vi "ConfigCreateProgram.vi"(11 "singlePumpCycleRefreshRatio":dbl) -> (3 "ProgramStopped":bool)   [LabVIEW 2018, in "Config.lvlib"]
uses:
  Config.lvlib
  <vilib>/xml/NI_XML.lvlib
  <vilib>/xml/Close Reference(Node).vi
  <vilib>/xml/Load XML File.vi
panel:
  in  "error in":errorcluster
  in  "Calc Minimal Acqu time":bool
  out "Minimal Acquisition Time":timestamp format="%<%H:%M:%S%3u>T"
  in  "stop":bool
  out "Loop Microscope Settings":string[][](array[string])
  out "Positions":string[][](array[string])
  out "Micro Ok?":bool
  out "Pos Ok?":bool
  in  "Load Microscope Settings":path
  in  "Load Positions":path
  in  "Acquire":bool
  in  "Load old Prog":bool
  out "error out":errorcluster
  in  "Clear":bool
  in  "Save":bool
  in  "Loop End":bool
  in  "Loop Start":bool
  in  "Incubate":bool
  in  "Change Reagent":bool
  in  "Feed":bool
  in  "Pump":bool
  out "Program Steps":i32[](listbox)
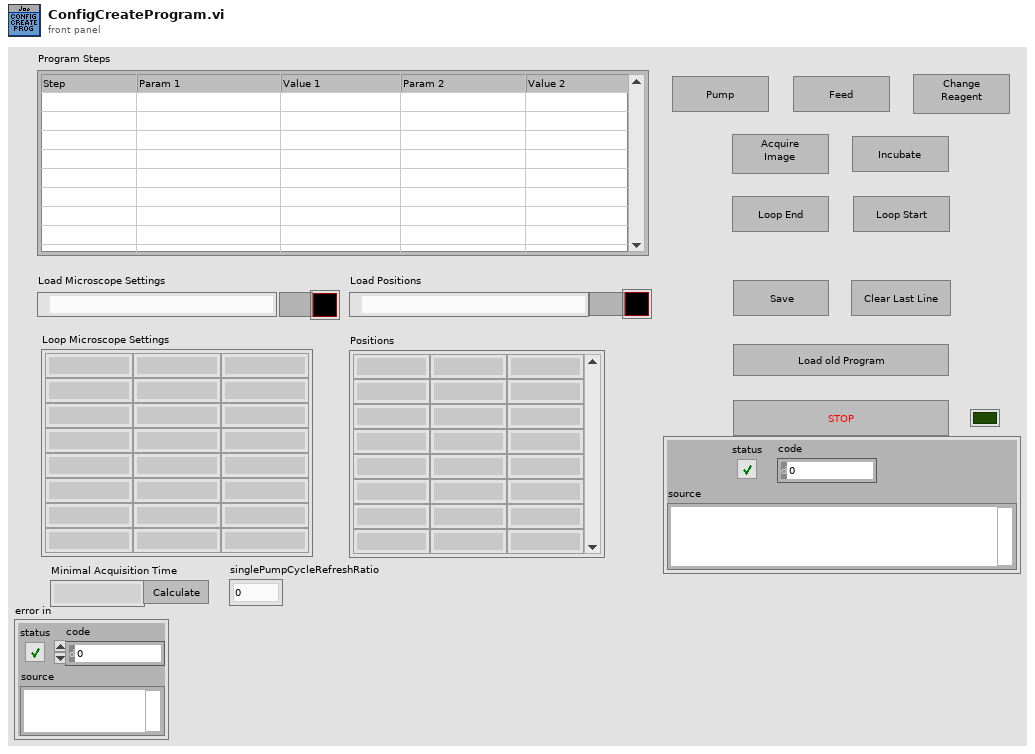
[diagram p1: front panel]
types:
  T1 = enum16{"open", "replace", "create", "open or create", "replace or create", "replace or create with confirmation"}
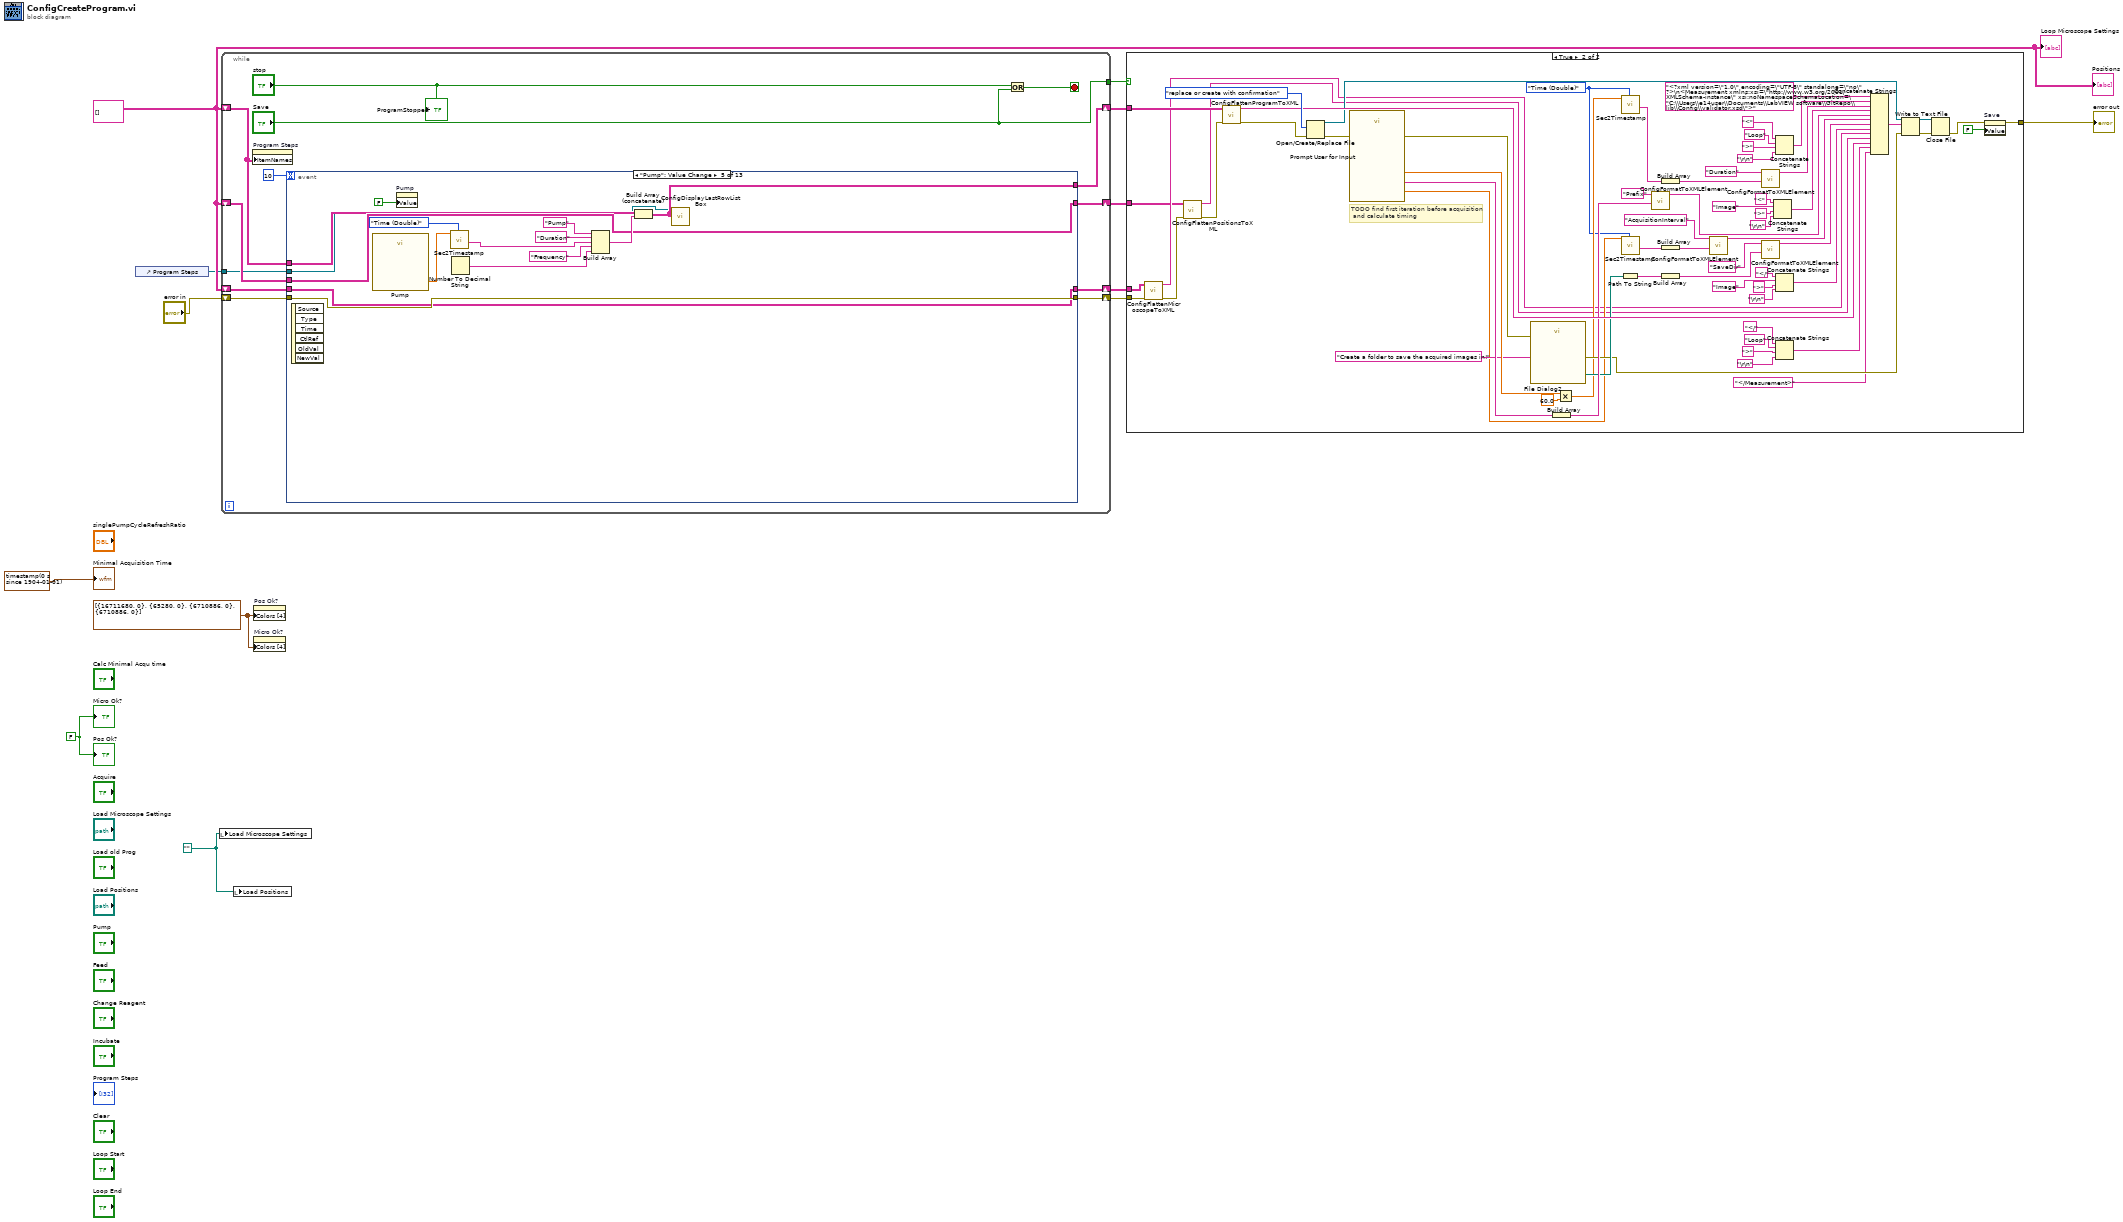
[diagram p0: block diagram]
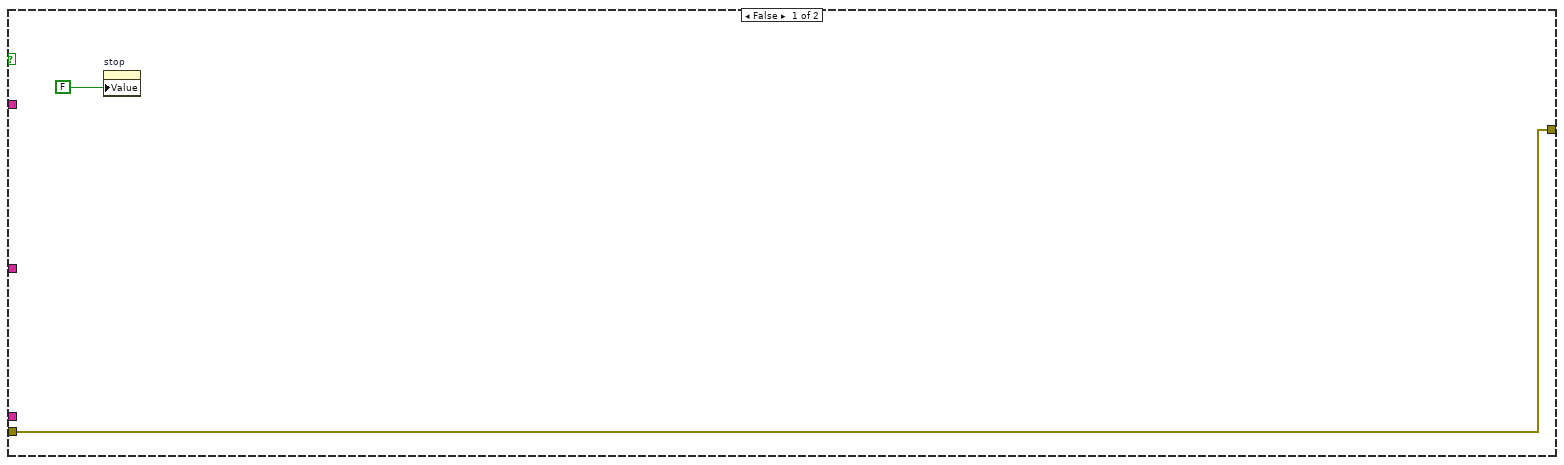
[diagram p2: hidden frame]
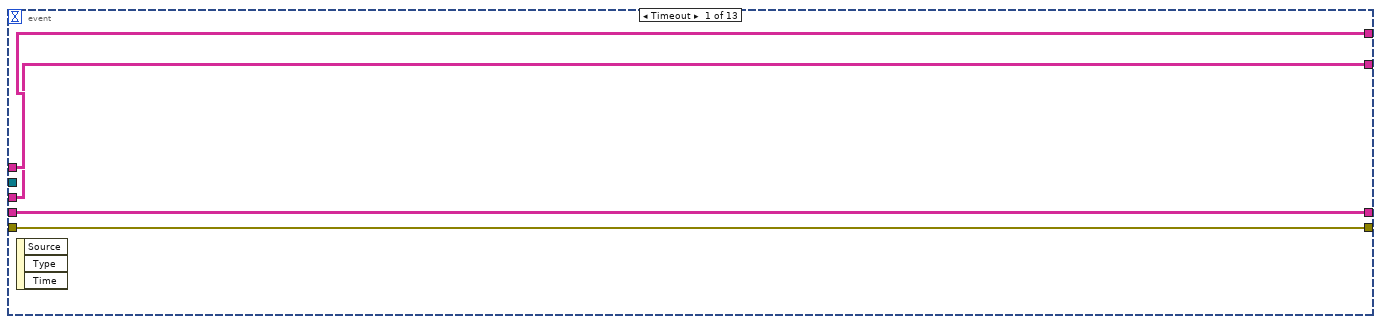
[diagram p3: hidden frame]
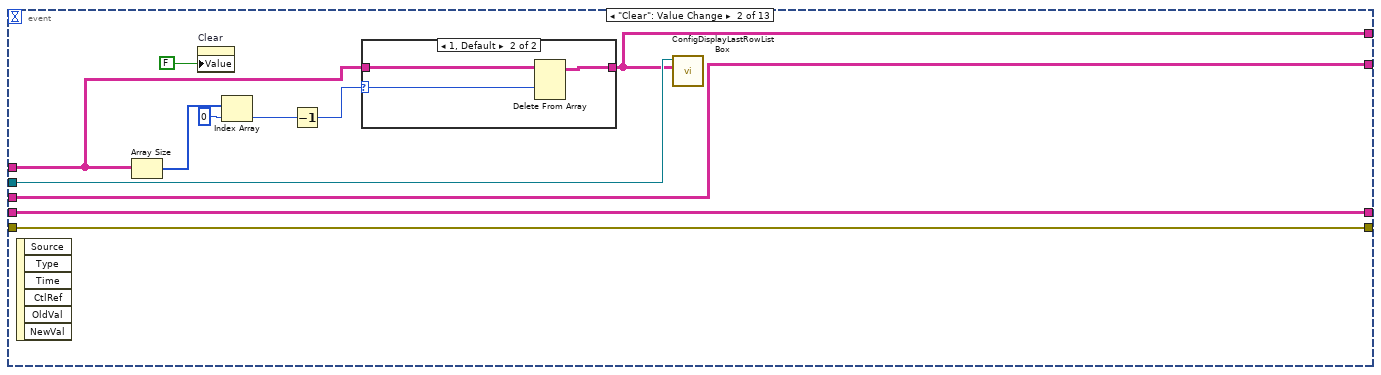
[diagram p4: hidden frame]
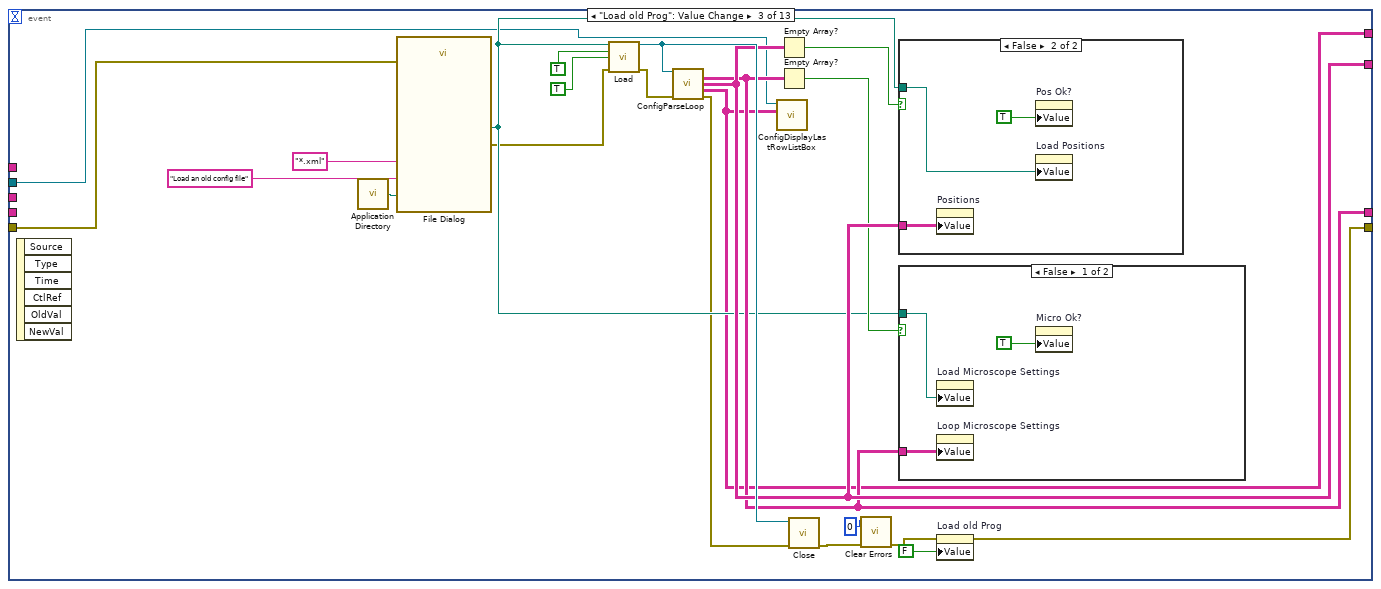
[diagram p6: hidden frame]
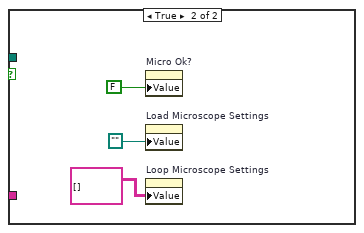
[diagram p7: hidden frame]
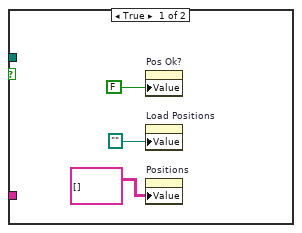
[diagram p8: hidden frame]
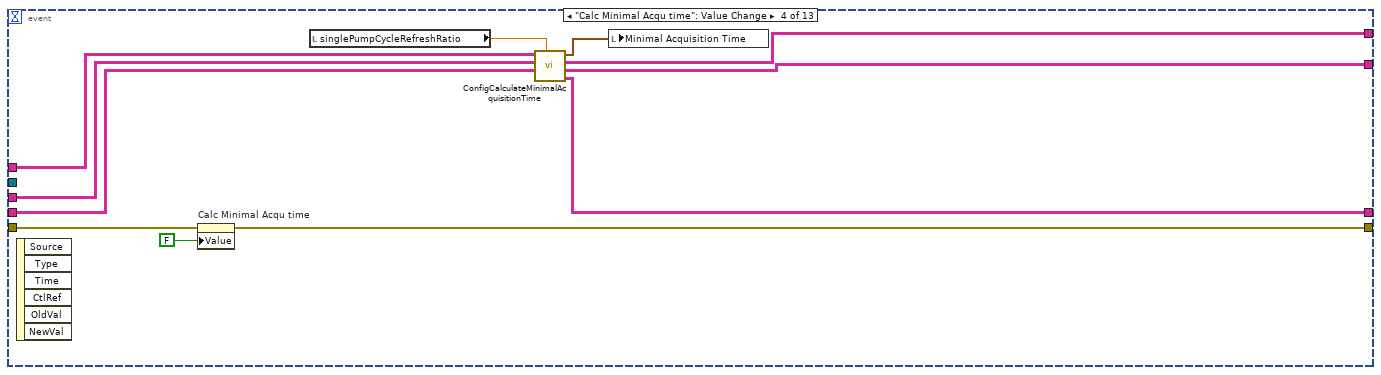
[diagram p9: hidden frame]
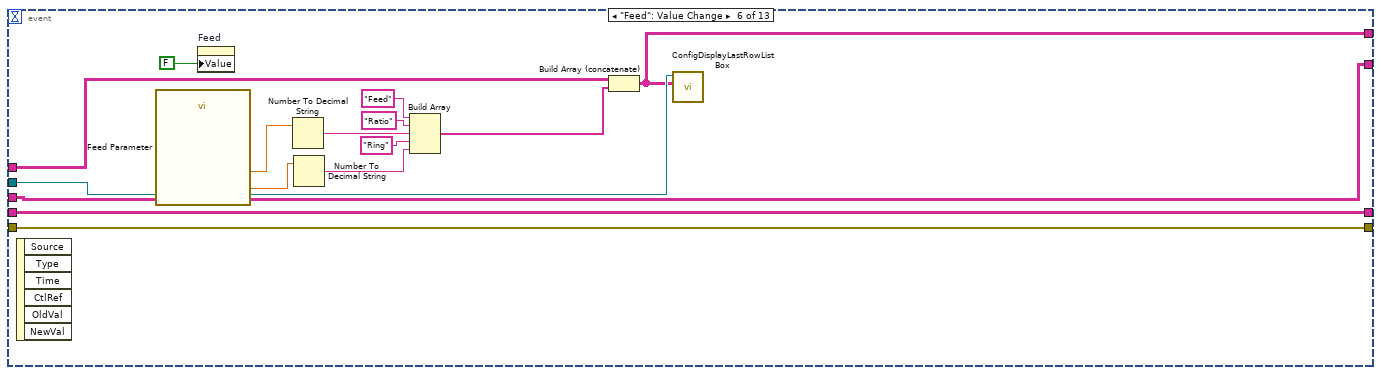
[diagram p10: hidden frame]
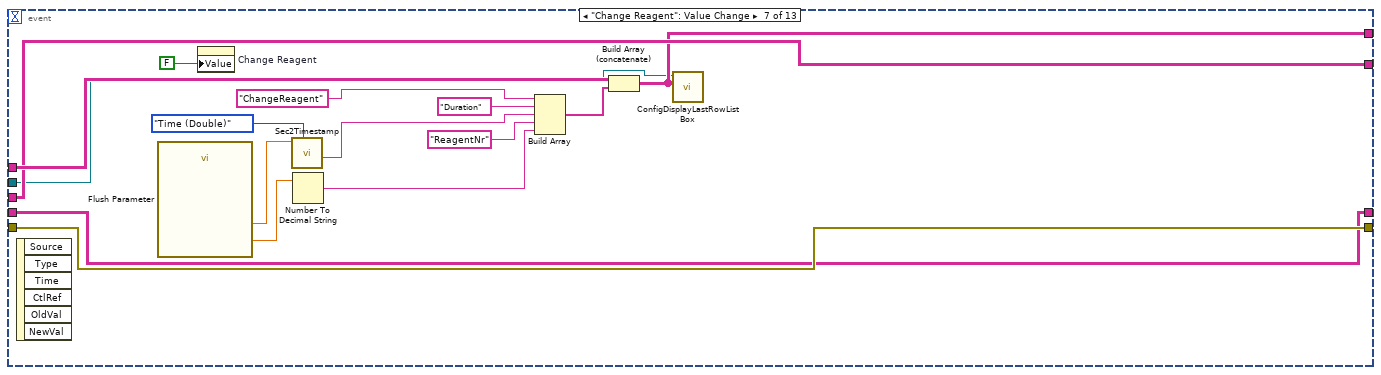
[diagram p11: hidden frame]
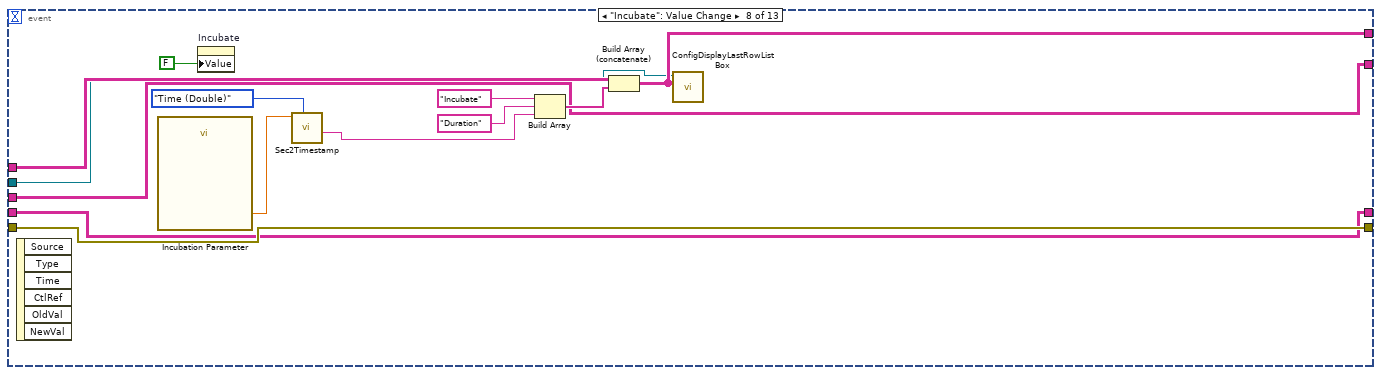
[diagram p12: hidden frame]
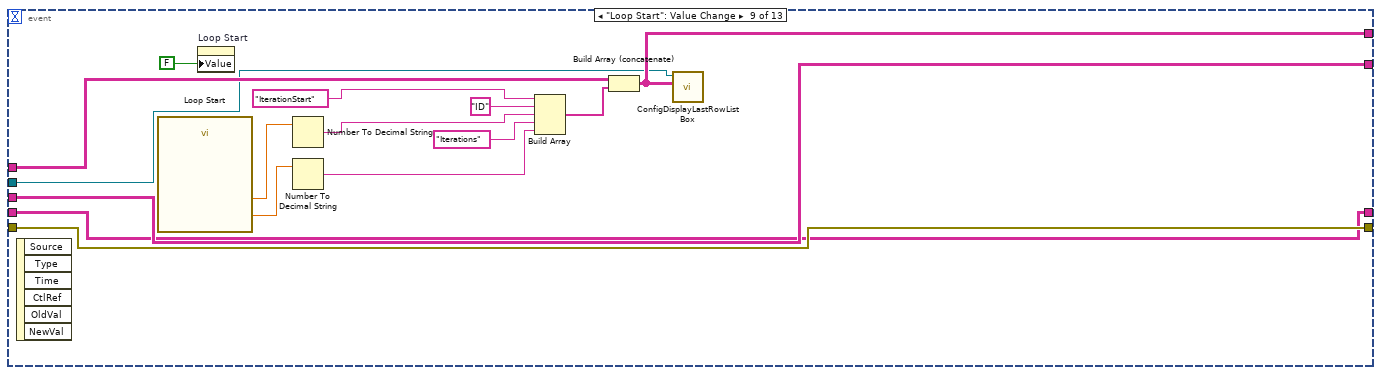
[diagram p13: hidden frame]
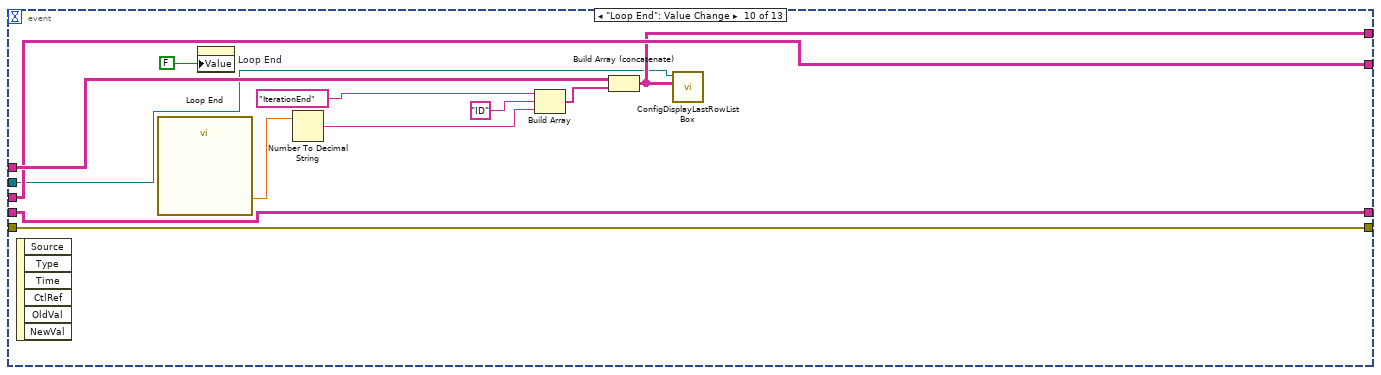
[diagram p14: hidden frame]
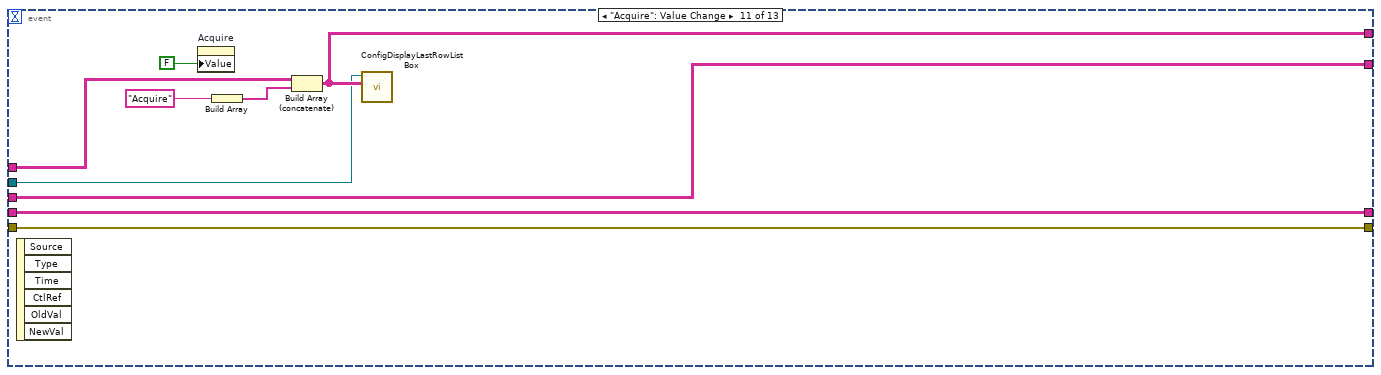
[diagram p15: hidden frame]
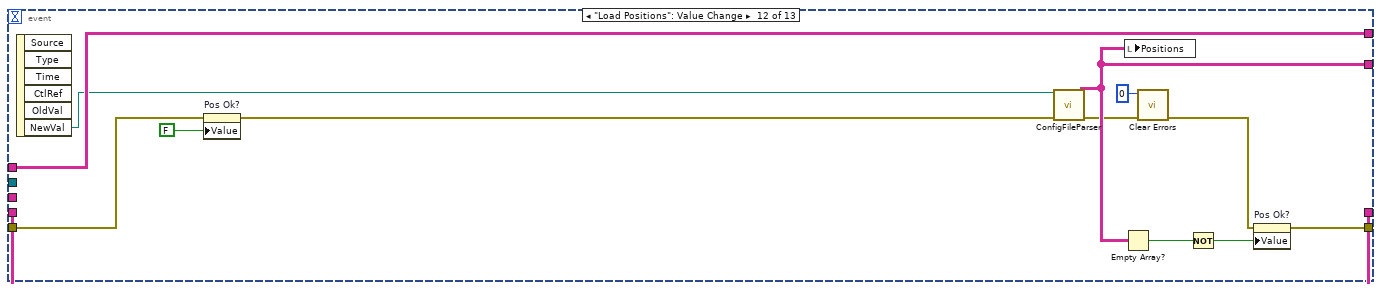
[diagram p16: hidden frame]
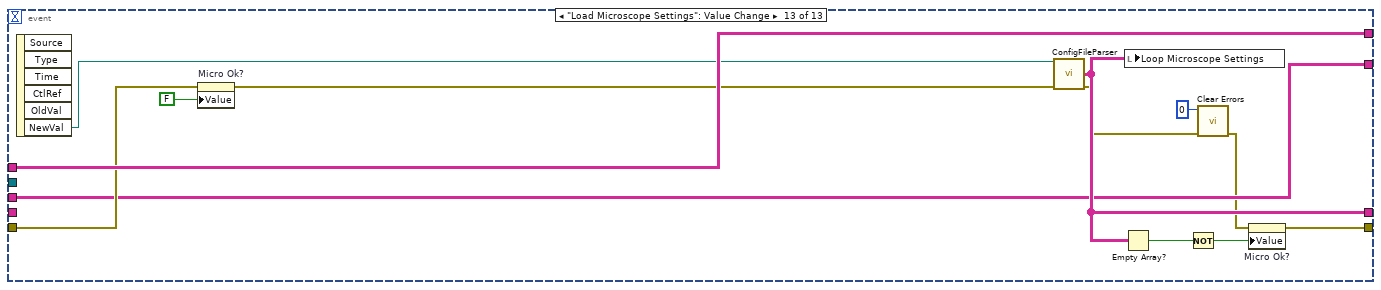
[diagram p17: hidden frame]
diagram:
  w2 = FALSE
  w3 = path ""
  w6 = string[][] [] ("ItemNames")
  w11 = cluster{u32, u32}[] [{16711680, 0}, {65280, 0}, {6710886, 0}, {6710886, 0}] ("Colors [4]")
  n1 = control-ref of="Program Steps"() -> (w5:refnum<vi>)
  n2 = local write "Load Microscope Settings"(w3) -> ()
  n3 = while {
    shift-right: [w26] -> w12
    shift-left: w6 -> [w22]
    shift-right: [w23] -> w9
    shift-left: "error in" -> [w24]
    shift-right: [w19] -> w7
    shift-left: w6 -> [w18]
    shift-right: [w20] -> w10
    shift-left: w6 -> [w21]
    tunnel: ["Save"] -> w8
    tunnel: w5 -> [w14]
    stop <- w17 stop-if-true
    n4 = property on="Program Steps" class="MCListbox (strict)"("ItemNames"=w22) -> ()  [unwired: 2 in, 2 out]
    n5 = event shown="[4] \"Pump\": Value Change" {
      selector: _ -> [_ _ _ _ _ _ _ _ _ _ _ _ _]
      dyn-events: _ -> [_ _ _ _ _ _ _ _ _ _ _ _ _]
      timeout: 10 -> [_ _ _ _ _ _ _ _ _ _ _ _ _]
      tunnel: w22 -> [w30 w41 _ w85 w95 w117 w133 w147 w161 w174 w185 w198 w211]
      tunnel: [w30 w31 w52 w80 w92 w109 w122 w138 w151 w166 w178 w198 w211] -> w26
      tunnel: w24 -> [w29 w35 w61 w88 w99 w113 w128 w144 w154 w169 w181 w193 w206]
      tunnel: [w29 w35 w54 w90 w99 w113 w128 w144 w154 w169 w181 w192 w205] -> w23
      tunnel: [w28 w34 w58 w81 w98 w112 w127 w143 w153 w168 w180 w191 w203] -> w19
      tunnel: w21 -> [w27 w33 _ w83 w97 w111 w126 w142 w152 w167 w179 w190 _]
      tunnel: [w27 w33 w56 w82 w97 w111 w126 w142 w152 w167 w179 w190 w204] -> w20
      tunnel: w18 -> [w28 w34 _ w84 w98 w112 w127 w143 w153 w168 w180 _ w203]
      tunnel: w14 -> [_ w32 w53 _ w91 w110 w121 w137 w150 w165 w177 _ _]
      event Timeout {
        n6 = event-data() -> ()  [unwired: 1 in, 3 out]
      }
      event "Clear": Value Change {
        n7 = event-data() -> ()  [unwired: 1 in, 6 out]
        n8 = Array Size(array=w41) -> (size(s)=w40:i32[])
        n9 = property on="Clear" class="Bool (strict)"("Value"=FALSE ("Value (Signaling)")) -> ()  [unwired: 2 in, 2 out]
        n10 = Index Array(array=w40, index=0) -> (element=w38:i32)
        n11 = Decrement(x=w38) -> (x-1=w37:i32)
        n12 = case shown="1, Default" w37 {
          selector: w37 -> [_ w43]
          tunnel: [w42 w45] -> w31
          tunnel: w41 -> [w42 w44]
          frame -1 {
          }
          frame 1, Default {
            n13 = Delete From Array(array=w44, index (row)=w43) -> (array with subset deleted=w45:string[][])  [unwired: 2 in, 1 out]
          }
        }
        n14 = call "ConfigDisplayLastRowListBox.vi"("Array"=w31, "reference"=w32) -> ()  [unwired: 10 in]
      }
      event "Load old Prog": Value Change {
        n15 = event-data() -> ()  [unwired: 1 in, 6 out]
        n16 = call <vilib>:"Application Directory.vi"() -> ("Application Directory"=w64:path)
        n17 = call "File Dialog"("start path"=w64, "prompt"="Load an old config file", "error in"=w61, "pattern label"="*.xml") -> ("selected path"=w55:path, "error out"=w49:errorcluster)  [unwired: 8 in, 2 out]
        n18 = call-poly <vilib>:"Load.vi"("path to XML document"=w55, "process namespaces (False)"=TRUE, "process schema (False)"=TRUE, "error in (no error)"=w49) -> ("DOM document out"=w60:refnum<k20>, "error out"=w50:errorcluster)  [unwired: 9 in, 1 out]
        n19 = call "ConfigParseLoop.vi"("Root Refnum in"=w60, "error in (no error)"=w50) -> ("Loop Microscope Settings"=w56:string[][], "Position Settings"=w58:string[][], "Program"=w52:string[][], "error out"=w51:errorcluster)  [unwired: 9 in, 1 out]
        n20 = call "ConfigDisplayLastRowListBox.vi"("Array"=w52, "reference"=w53) -> ()  [unwired: 10 in]
        n21 = Empty Array?(array=w58) -> (empty?=w59:bool)
        n22 = Empty Array?(array=w56) -> (empty?=w57:bool)
        n23 = call-poly <vilib>:"Close.vi"("error in (no error)"=w51, "node"=w60) -> ("error out"=w47:errorcluster)  [unwired: 7 in]
        n24 = call <vilib>:"Clear Errors.vi"("error in (no error)"=w47, "specific error code to clear (0: all)"=0) -> ("error out"=w46:errorcluster)  [unwired: 4 in, 1 out]
        n25 = case shown="False" w59 {
          tunnel: w58 -> [_ w79]
          tunnel: w55 -> [_ w78]
          frame True {
            n26 = property on="Pos Ok?" class="Bool (strict)"("Value"=FALSE ("Pos Ok?")) -> ()  [unwired: 2 in, 2 out]
            n27 = property on="Load Positions" class="Path"("Value"=path "") -> ()  [unwired: 2 in, 2 out]
            n28 = property on="Positions" class="Arr (strict)"("Value"=string[][] []) -> ()  [unwired: 2 in, 2 out]
          }
          frame False {
            n29 = property on="Positions" class="Arr (strict)"("Value"=w79) -> ()  [unwired: 2 in, 2 out]
            n30 = property on="Pos Ok?" class="Bool (strict)"("Value"=TRUE ("Pos Ok?")) -> ()  [unwired: 2 in, 2 out]
            n31 = property on="Load Positions" class="Path"("Value"=w78) -> ()  [unwired: 2 in, 2 out]
          }
        }
        n32 = case shown="False" w57 {
          tunnel: w56 -> [w70 _]
          tunnel: w55 -> [w69 _]
          frame False {
            n33 = property on="Load Microscope Settings" class="Path"("Value"=w69) -> ()  [unwired: 2 in, 2 out]
            n34 = property on="Loop Microscope Settings" class="Arr (strict)"("Value"=w70) -> ()  [unwired: 2 in, 2 out]
            n35 = property on="Micro Ok?" class="Bool (strict)"("Value"=TRUE ("Micro Ok?")) -> ()  [unwired: 2 in, 2 out]
          }
          frame True {
            n36 = property on="Micro Ok?" class="Bool (strict)"("Value"=FALSE ("Micro Ok?")) -> ()  [unwired: 2 in, 2 out]
            n37 = property on="Load Microscope Settings" class="Path"("Value"=path "") -> ()  [unwired: 2 in, 2 out]
            n38 = property on="Loop Microscope Settings" class="Arr (strict)"("Value"=string[][] []) -> ()  [unwired: 2 in, 2 out]
          }
        }
        n39 = property on="Load old Prog" class="Bool (strict)"(error in=w46, "Value"=FALSE ("Value (Signaling)")) -> (error out=w54:errorcluster)  [unwired: 1 in, 1 out]
      }
      event "Calc Minimal Acqu time": Value Change {
        n40 = event-data() -> ()  [unwired: 1 in, 6 out]
        n41 = property on="Calc Minimal Acqu time" class="Bool (strict)"(error in=w88, "Value"=FALSE ("Calc Minimal Acqu time")) -> (error out=w90:errorcluster)  [unwired: 1 in, 1 out]
        n42 = local read "singlePumpCycleRefreshRatio"() -> (w86:dbl)
        n43 = call "ConfigCalculateMinimalAcquisitionTime.vi"("Single Pump Cycle Refresh Ratio"=w86, "Loop Microscope Settings"=w83, "Positions"=w84, "Program"=w85) -> ("Microscope Out"=w82:string[][], "Positions out"=w81:string[][], "Program out"=w80:string[][], "Time (Time Stamp)"=w87:timestamp)  [unwired: 4 in]
        n44 = local write "Minimal Acquisition Time"(w87) -> ()
      }
      event "Pump": Value Change {
        n45 = event-data() -> ()  [unwired: 1 in, 6 out]
        n46 = call "Pump"() -> ("Duration [s] (@ 4Hz)"=w96:dbl)  [unwired: 17 in, 2 out]
        n47 = property on="Pump" class="Bool (strict)"("Value"=FALSE ("Value (Signaling)")) -> ()  [unwired: 2 in, 2 out]
        n48 = call "Sec2Timestamp.vi"("Input Selection"=enum32{"Time (Double)", "Time (Time Stamp)"}."Time (Double)", "Input Time (Double)"=w96) -> ("time string"=w93:string)  [unwired: 7 in, 2 out]
        n49 = Number To Decimal String() -> (decimal integer string=w102:string)  [unwired: 2 in]
        n50 = Build Array("Pump", "Duration", w93, "Frequency", w102) -> (w104:string[])
        n51 = Build Array (concatenate)(w95, w104) -> (w92:string[][])
        n52 = call "ConfigDisplayLastRowListBox.vi"("Array"=w92, "reference"=w91) -> ()  [unwired: 10 in]
      }
      event "Feed": Value Change {
        n53 = event-data() -> ()  [unwired: 1 in, 6 out]
        n54 = call "Feed Parameter"() -> ("Ring"=w108:dbl, "Ratio [%]"=w119:dbl)  [unwired: 16 in, 2 out]
        n55 = property on="Feed" class="Bool (strict)"("Value"=FALSE ("Value (Signaling)")) -> ()  [unwired: 2 in, 2 out]
        n56 = Number To Decimal String(number=w119) -> (decimal integer string=w115:string)  [unwired: 1 in]
        n57 = Number To Decimal String(number=w108) -> (decimal integer string=w107:string)  [unwired: 1 in]
        n58 = Build Array("Feed", "Ratio", w115, "Ring" ("element"), w107) -> (w118:string[])
        n59 = Build Array (concatenate)(w117, w118) -> (w109:string[][])
        n60 = call "ConfigDisplayLastRowListBox.vi"("Array"=w109, "reference"=w110) -> ()  [unwired: 10 in]
      }
      event "Change Reagent": Value Change {
        n61 = event-data() -> ()  [unwired: 1 in, 6 out]
        n62 = call "Flush Parameter"() -> ("Flush Duration [s]"=w125:dbl, "Reagent Nr."=w130:dbl)  [unwired: 16 in, 2 out]
        n63 = property on="Change Reagent" class="Bool (strict)"("Value"=FALSE ("Value (Signaling)")) -> ()  [unwired: 2 in, 2 out]
        n64 = call "Sec2Timestamp.vi"("Input Selection"=enum32{"Time (Double)", "Time (Time Stamp)"}."Time (Double)", "Input Time (Double)"=w125) -> ("time string"=w123:string)  [unwired: 7 in, 2 out]
        n65 = Number To Decimal String(number=w130) -> (decimal integer string=w129:string)  [unwired: 1 in]
        n66 = Build Array("ChangeReagent", "Duration", w123, "ReagentNr", w129) -> (w134:string[])
        n67 = Build Array (concatenate)(w133, w134) -> (w122:string[][])
        n68 = call "ConfigDisplayLastRowListBox.vi"("Array"=w122, "reference"=w121) -> ()  [unwired: 10 in]
      }
      event "Incubate": Value Change {
        n69 = event-data() -> ()  [unwired: 1 in, 6 out]
        n70 = call "Incubation Parameter"() -> ("Duration [s]"=w141:dbl)  [unwired: 17 in, 2 out]
        n71 = property on="Incubate" class="Bool (strict)"("Value"=FALSE ("Value (Signaling)")) -> ()  [unwired: 2 in, 2 out]
        n72 = call "Sec2Timestamp.vi"("Input Selection"=enum32{"Time (Double)", "Time (Time Stamp)"}."Time (Double)", "Input Time (Double)"=w141) -> ("time string"=w139:string)  [unwired: 7 in, 2 out]
        n73 = Build Array("Incubate", "Duration", w139) -> (w148:string[])
        n74 = Build Array (concatenate)(w147, w148) -> (w138:string[][])
        n75 = call "ConfigDisplayLastRowListBox.vi"("Array"=w138, "reference"=w137) -> ()  [unwired: 10 in]
      }
      event "Loop Start": Value Change {
        n76 = event-data() -> ()  [unwired: 1 in, 6 out]
        n77 = call "Loop Start"() -> ("ID"=w159:dbl, "Iterations"=w163:dbl)  [unwired: 16 in, 2 out]
        n78 = property on="Loop Start" class="Bool (strict)"("Value"=FALSE ("Value (Signaling)")) -> ()  [unwired: 2 in, 2 out]
        n79 = Number To Decimal String(number=w159) -> (decimal integer string=w158:string)  [unwired: 1 in]
        n80 = Number To Decimal String(number=w163) -> (decimal integer string=w155:string)  [unwired: 1 in]
        n81 = Build Array("IterationStart", "ID" ("element"), w158, "Iterations", w155) -> (w162:string[])
        n82 = Build Array (concatenate)(w161, w162) -> (w151:string[][])
        n83 = call "ConfigDisplayLastRowListBox.vi"("Array"=w151, "reference"=w150) -> ()  [unwired: 10 in]
      }
      event "Loop End": Value Change {
        n84 = event-data() -> ()  [unwired: 1 in, 6 out]
        n85 = call "Loop End"() -> ("ID"=w172:dbl)  [unwired: 17 in, 2 out]
        n86 = property on="Loop End" class="Bool (strict)"("Value"=FALSE ("Value (Signaling)")) -> ()  [unwired: 2 in, 2 out]
        n87 = Number To Decimal String(number=w172) -> (decimal integer string=w171:string)  [unwired: 1 in]
        n88 = Build Array("IterationEnd", "ID" ("element"), w171) -> (w175:string[])
        n89 = Build Array (concatenate)(w174, w175) -> (w166:string[][])
        n90 = call "ConfigDisplayLastRowListBox.vi"("Array"=w166, "reference"=w165) -> ()  [unwired: 10 in]
      }
      event "Acquire": Value Change {
        n91 = event-data() -> ()  [unwired: 1 in, 6 out]
        n92 = property on="Acquire" class="Bool (strict)"("Value"=FALSE ("Value (Signaling)")) -> ()  [unwired: 2 in, 2 out]
        n93 = Build Array("Acquire") -> (w182:string[])
        n94 = Build Array (concatenate)(w185, w182) -> (w178:string[][])
        n95 = call "ConfigDisplayLastRowListBox.vi"("Array"=w178, "reference"=w177) -> ()  [unwired: 10 in]
      }
      event "Load Positions": Value Change {
        n96 = event-data() -> ("NewVal"=w197:path)  [unwired: 1 in, 5 out]
        n97 = property on="Pos Ok?" class="Bool (strict)"(error in=w193, "Value"=FALSE) -> (error out=w188:errorcluster)  [unwired: 1 in, 1 out]
        n98 = call "ConfigFileParser.vi"("Path"=w197, "error in"=w188) -> ("Positions"=w191:string[][], "error out"=w189:errorcluster)  [unwired: 8 in, 4 out]
        n99 = Empty Array?(array=w191) -> (empty?=w195:bool)
        n100 = local write "Positions"(w191) -> ()
        n101 = call <vilib>:"Clear Errors.vi"("error in (no error)"=w189, "specific error code to clear (0: all)"=0) -> ("error out"=w187:errorcluster)  [unwired: 4 in, 1 out]
        n102 = Not(x=w195) -> (.not. x?=w196:bool)
        n103 = property on="Pos Ok?" class="Bool (strict)"(error in=w187, "Value"=w196) -> (error out=w192:errorcluster)  [unwired: 1 in, 1 out]
      }
      event "Load Microscope Settings": Value Change {
        n104 = event-data() -> ("NewVal"=w210:path)  [unwired: 1 in, 5 out]
        n105 = property on="Micro Ok?" class="Bool (strict)"(error in=w206, "Value"=FALSE) -> (error out=w199:errorcluster)  [unwired: 1 in, 1 out]
        n106 = call "ConfigFileParser.vi"("Path"=w210, "error in"=w199) -> ("Loop Microscope Settings"=w204:string[][], "error out"=w200:errorcluster)  [unwired: 8 in, 4 out]
        n107 = Empty Array?(array=w204) -> (empty?=w208:bool)
        n108 = local write "Loop Microscope Settings"(w204) -> ()
        n109 = Not(x=w208) -> (.not. x?=w209:bool)
        n110 = call <vilib>:"Clear Errors.vi"("error in (no error)"=w200, "specific error code to clear (0: all)"=0) -> ("error out"=w201:errorcluster)  [unwired: 4 in, 1 out]
        n111 = property on="Micro Ok?" class="Bool (strict)"(error in=w201, "Value"=w209) -> (error out=w205:errorcluster)  [unwired: 1 in, 1 out]
      }
    }
    n112 = Or(x="stop", y="Save") -> (x .or. y?=w17:bool)
    "ProgramStopped" <- "stop"
  }
  n113 = local write "Load Positions"(w3) -> ()
  n114 = property on="Pos Ok?" class="Bool (strict)"("Colors [4]"=w11) -> ()  [unwired: 2 in, 2 out]
  n115 = property on="Micro Ok?" class="Bool (strict)"("Colors [4]"=w11) -> ()  [unwired: 2 in, 2 out]
  n116 = case shown="True" w8 {
    tunnel: [w213 w278] -> w13
    tunnel: w12 -> [_ w275]
    tunnel: w10 -> [_ w214]
    tunnel: w9 -> [w213 w235]
    tunnel: w7 -> [_ w215]
    frame False {
      n117 = property on="stop" class="Bool (strict)"("Value"=FALSE ("stop")) -> ()  [unwired: 2 in, 2 out]
    }
    frame True {
      w220 = enum32{"Time (Double)", "Time (Time Stamp)"}."Time (Double)" ("Input Selection")
      # "TODO find first iteration before acquisition\n and calculate timing"
      n118 = call "ConfigFlattenMicroscopeToXML.vi"("error in (no error)"=w235, "MicroscopeArray"=w214) -> ("error out"=w217:errorcluster, "MicrosocopeXML"=w219:string)  [unwired: 8 in]
      n119 = call "ConfigFlattenPositionsToXML.vi"("error in"=w217, "Position Array in"=w215) -> ("error out"=w216:errorcluster, "Position XML"=w218:string)  [unwired: 8 in]
      n120 = call "ConfigFlattenProgramToXML.vi"("error in (no error)"=w216, "ProgramArray"=w275) -> ("error out"=w254:errorcluster, "ProgramXML"=w263:string)  [unwired: 8 in]
      n121 = Open/Create/Replace File(error in=w254, operation (0:open)=T1."replace or create with confirmation") -> (refnum out=w250:refnum<file>, error out=w253:errorcluster)  [unwired: 4 in, 1 out]
      n122 = call "Prompt User for Input"("error in (no error)"=w253) -> ("File Prefix"=w245:string, "Total Acquisition Time [min]"=w267:dbl, "Acquisition Interval [s]"=w223:dbl, "error out"=w232:errorcluster)  [unwired: 14 in, 1 out]
      n123 = call "File Dialog2"("prompt"="Create a folder to save the acquired images in!" ("prompt (Create Folder)"), "error in"=w232) -> ("selected path"=w233:path, "error out"=w231:errorcluster)  [unwired: 10 in, 2 out]
      n124 = Build Array(w245) -> (w244:string[])
      n125 = Multiply(x=w267, y=60.0) -> (x*y=w225:dbl)
      n126 = Path To String(path=w233) -> (string=w241:string)
      n127 = call "Sec2Timestamp.vi"("Input Selection"=w220, "Input Time (Double)"=w225) -> ("time string"=w224:string)  [unwired: 7 in, 2 out]
      n128 = call "Sec2Timestamp.vi"("Input Selection"=w220, "Input Time (Double)"=w223) -> ("time string"=w222:string)  [unwired: 7 in, 2 out]
      n129 = call "ConfigFormatToXMLElement.vi"("Value"=w244, "outer Tag"="Prefix" ("string")) -> ("Resulting String"=w243:string)  [unwired: 9 in]
      n130 = Build Array(w224) -> (w237:string[])
      n131 = Build Array(w222) -> (w221:string[])
      n132 = Build Array(w241) -> (w240:string[])
      n133 = call "ConfigFormatToXMLElement.vi"("Value"=w221, "outer Tag"="AcquisitionInterval" ("string")) -> ("Resulting String"=w248:string)  [unwired: 9 in]
      n134 = call "ConfigFormatToXMLElement.vi"("Value"=w237, "outer Tag"="Duration" ("string")) -> ("Resulting String"=w236:string)  [unwired: 9 in]
      n135 = call "ConfigFormatToXMLElement.vi"("Value"=w240, "outer Tag"="SaveDir" ("string")) -> ("Resulting String"=w239:string)  [unwired: 9 in]
      n136 = Concatenate Strings("<" ("string"), "Image" ("string"), ">" ("string"), "\r\n") -> (w265:string)
      n137 = Concatenate Strings("<" ("string"), "Loop" ("string"), ">" ("string"), "\r\n") -> (w260:string)
      n138 = Concatenate Strings("</" ("string"), "Image" ("string"), ">" ("string"), "\r\n") -> (w264:string)
      n139 = Concatenate Strings("</" ("string"), "Loop" ("string"), ">" ("string"), "\r\n") -> (w256:string)
      n140 = Concatenate Strings("<?xml version=\"1.0\" encoding=\"UTF-8\" standalone=\"no\" ?>\n<Measurement xmlns:xsi=\"http://www.w3.org/2001/XMLSchema-instance\" xsi:noNamespaceSchemaLocation=\"C:\\Users\\e14user\\Documents\\LabVIEW software\\GitRepo\\lib\\Config\\validator.xsd\">", w260, w236, w265, w243, w248, w239, w264, w219, w218, w263, w256, "</Measurement>" ("string")) -> (w249:string)
      n141 = Write to Text File(file (use dialog)=w250, text=w249, error in=w231) -> (refnum out=w251:refnum<file>, error out=w252:errorcluster)  [unwired: 1 in, 1 out]
      n142 = Close File(refnum=w251, error in=w252) -> (error out=w277:errorcluster)  [unwired: 1 out]
      n143 = property on="Save" class="Bool (strict)"(error in=w277, "Value"=FALSE ("Save")) -> (error out=w278:errorcluster)  [unwired: 1 in, 1 out]
    }
  }
  "error out" <- w13
  "Pos Ok?" <- w2
  "Micro Ok?" <- w2
  "Positions" <- w6
  "Loop Microscope Settings" <- w6
  "Minimal Acquisition Time" <- timestamp(0 s since 1904-01-01)
